vi "20170516-lecture4-2 prof ProducerConsumerQueue.vi"() -> ()   [LabVIEW 2014]
doc: "Use this template to build a producer/consumer design pattern. Use this template when you need to execute a process, such as data analysis, when a data source, such as a triggered acquisition, produces data at an uneven rate and you need to execute the process when the data becomes available."
panel:
  out "Queue Backlog":i32(slide) scale=0.0..100.0
  in  "Wait(ms) in Consumer Loop":u32(slide) scale=0.0..10000.0
  out "Dequeued Data":string="element"
  in  "Data to Enqueue":string="element"
  in  "Enqueue Data":bool
  in  "stop":bool
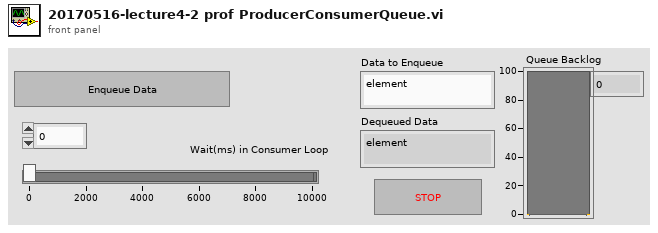
[diagram p1: front panel]
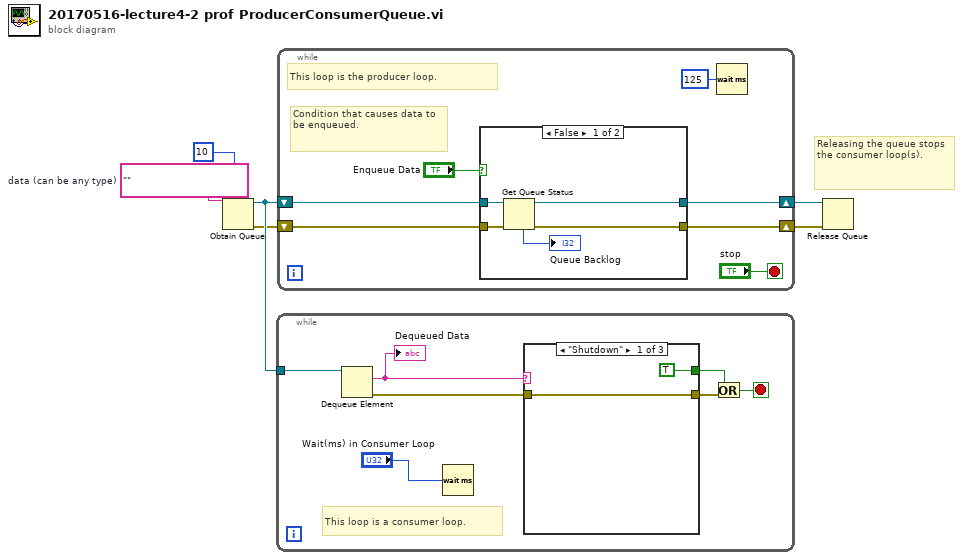
[diagram p0: block diagram]
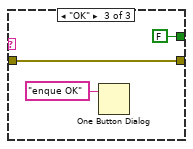
[diagram p3: hidden frame]
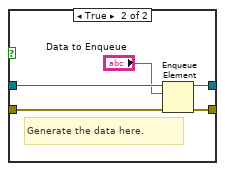
[diagram p4: hidden frame]
diagram:
  w2 = ""  # data (can be any type)
  # "Releasing the queue stops the consumer loop(s)."
  n1 = Obtain Queue(max queue size (-1, unlimited)=10, element data type=w2) -> (queue out=w6:refnum<queue>, error out=w5:errorcluster)  [unwired: 3 in, 1 out]
  n2 = while {
    tunnel: w6 -> [w13]
    stop <- w10 stop-if-true
    # "This loop is a consumer loop."
    n3 = Dequeue Element(queue=w13) -> (element=w7:string, error out=w12:errorcluster)  [unwired: 2 in, 2 out]
    "Dequeued Data" <- w7
    n4 = Wait (ms)(milliseconds to wait="Wait(ms) in Consumer Loop") -> ()  [unwired: 1 out]
    n5 = case shown="\"Shutdown\"" w7 {
      tunnel: [TRUE _ FALSE] -> w9
      tunnel: [w14 w16 w18] -> w11
      tunnel: w12 -> [w14 w16 w18]
      frame "Shutdown" {
      }
      frame Default {
      }
      frame "OK" {
        n6 = One Button Dialog(message="enque OK") -> ()  [unwired: 1 in, 1 out]
      }
    }
    n7 = Or(x=w9, y=w11) -> (x .or. y?=w10:bool)
  }
  n8 = while {
    shift-right: [w22] -> w3
    shift-left: w5 -> [w23]
    shift-right: [w24] -> w4
    shift-left: w6 -> [w25]
    stop <- "stop" stop-if-true
    # "Condition that causes data to be enqueued."
    # "This loop is the producer loop."
    n9 = case shown="False" "Enqueue Data" {
      tunnel: w25 -> [w29 w36]
      tunnel: [w28 w35] -> w24
      tunnel: w23 -> [w31 w34]
      tunnel: [w30 w33] -> w22
      frame False {
        n10 = Get Queue Status(queue=w29, error in (no error)=w31) -> (queue out=w28:refnum<queue>, error out=w30:errorcluster, # elements in queue=→"Queue Backlog":i32)  [unwired: 1 in, 5 out]
      }
      frame True {
        # "Generate the data here."
        n11 = Enqueue Element(queue=w36, element="Data to Enqueue", error in (no error)=w34) -> (queue out=w35:refnum<queue>, error out=w33:errorcluster)  [unwired: 1 in, 1 out]
      }
    }
    n12 = Wait (ms)(milliseconds to wait=u32 125) -> ()  [unwired: 1 out]
  }
  n13 = Release Queue(queue=w4, error in (no error)=w3) -> ()  [unwired: 1 in, 3 out]
